vi "HW_6p1_Task2_weesesr.vi"() -> ()   [LabVIEW 2016]
panel:
  out "Number of Times Temp Exceeded 250C":dbl
  out "Average Temperature of Day":dbl
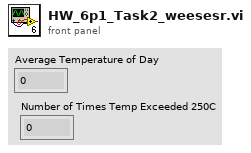
[diagram p1: front panel]
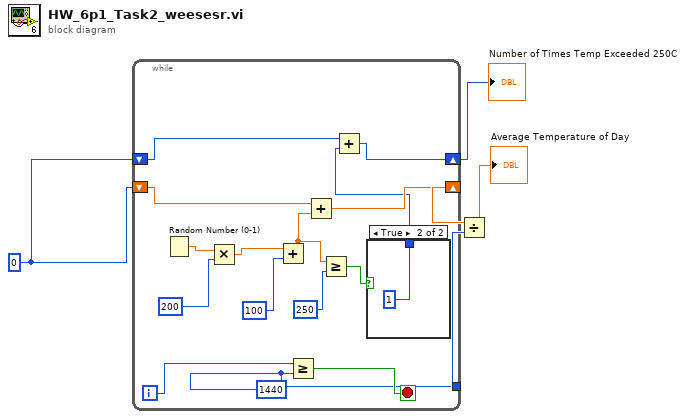
[diagram p0: block diagram]
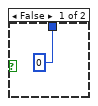
[diagram p2: hidden frame]
diagram:
  w2 = 0
  n1 = while {
    shift-right: [w13] -> w5
    shift-left: w2 -> [w14]
    tunnel: [w12] -> w4
    shift-right: [w7] -> w1
    shift-left: w2 -> [w8]
    i -> [w20]
    stop <- w19 stop-if-true
    w12 = 1440
    n2 = Random Number (0-1)() -> (number: 0 to 1=w18:dbl)
    n3 = Multiply(x=w18, y=200) -> (x*y=w15:dbl)
    n4 = Add(x=w15, y=100) -> (x+y=w11:dbl)
    n5 = Greater Or Equal?(x=w20, y=w12) -> (x >= y?=w19:bool)
    n6 = Add(x=w14, y=w11) -> (x+y=w13:dbl)
    n7 = Greater Or Equal?(x=w11, y=250) -> (x >= y?=w9:bool)
    n8 = case shown="True" w9 {
      tunnel: [0 1] -> w6
      frame False {
      }
      frame True {
      }
    }
    n9 = Add(x=w8, y=w6) -> (x+y=w7:i32)
  }
  "Number of Times Temp Exceeded 250C" <- w1
  n10 = Divide(x=w5, y=w4) -> (x/y=→"Average Temperature of Day":dbl)
